vi "DPT Parse Debug Log.vi"(10 "text":string) -> (1 "Headers for Data":string[](array[string]), 2 "Array [raw rod, filt rod, outlet t, inlet t, coil, curve or hr]":i32[][](array[numeric]), 3 "Time Array":string[](array[string]))   [LabVIEW 2016]
panel:
  out "Numeric":i32
  out "Fault":i32
  out "Coil":i32
  out "Data Line":bool
  out "Time":string
  out "Line":string
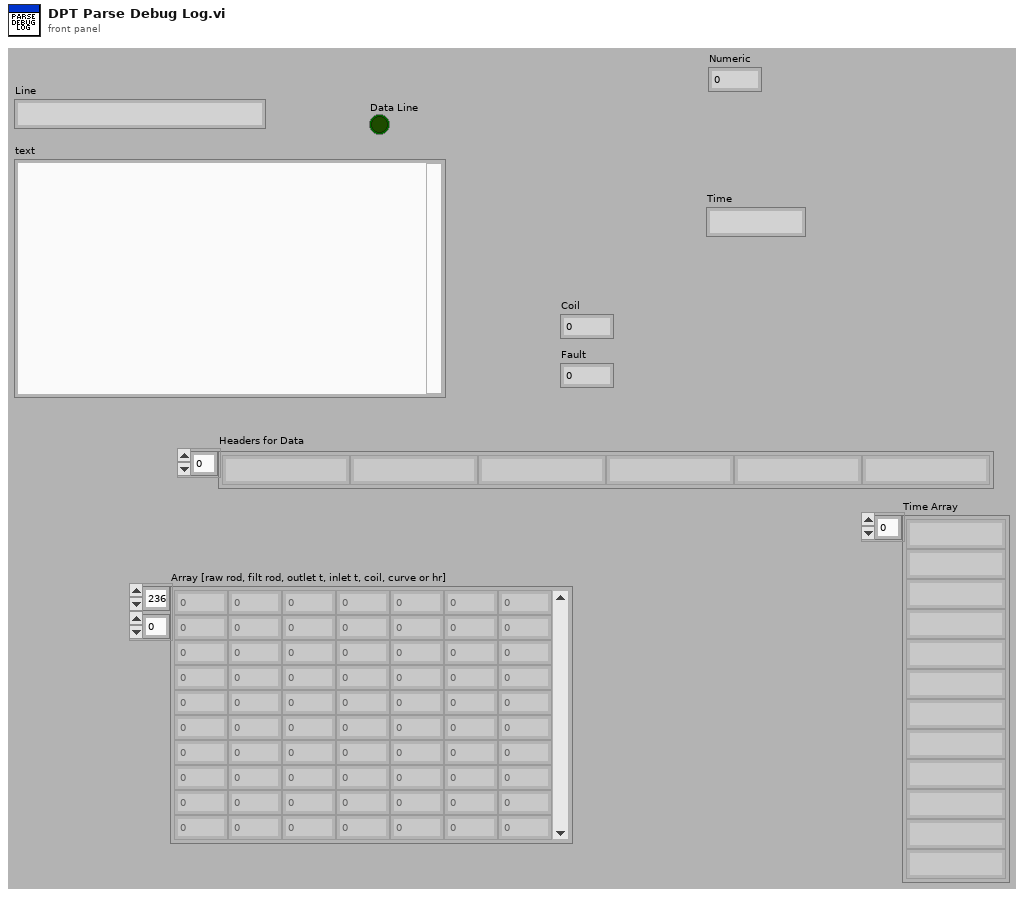
[diagram p1: front panel]
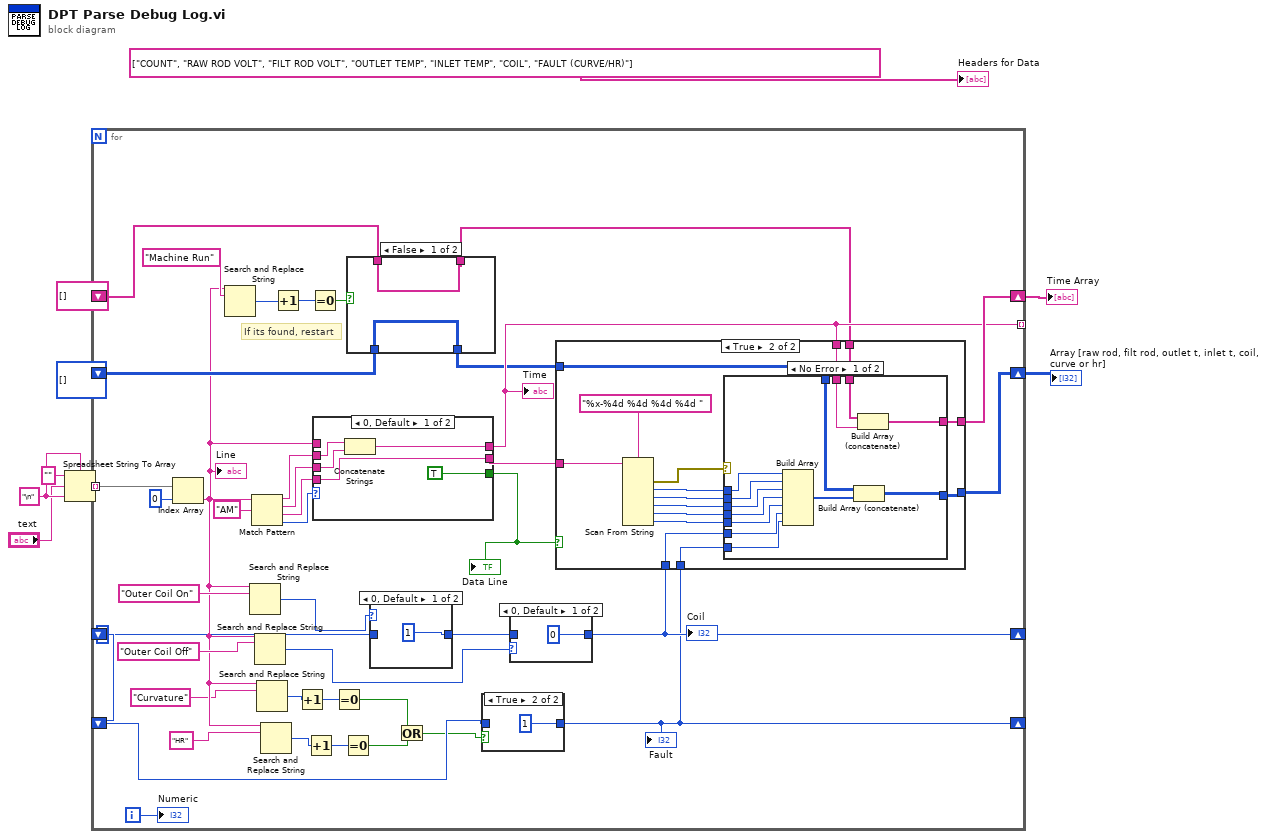
[diagram p0: block diagram]
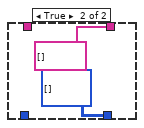
[diagram p5: hidden frame]
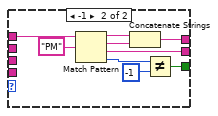
[diagram p8: hidden frame]
diagram:
  w4 = 0 ("output 5")
  w9 = "\n" ("delimiter (Tab)")
  n1 = Spreadsheet String To Array(delimiter (Tab)=w9, format string="", spreadsheet string="text", array type (2D Dbl)=w9) -> (array=w10:string[][])
  n2 = for {
    tunnel: w10 -> [w50] mode=indexing
    shift-right: [w11] -> w2
    shift-left: i32[][] [] -> [w34]
    tunnel: [w37] -> _ mode=indexing
    shift-right: [w38] -> w3
    shift-left: string[] [] -> [w32]
    shift-right: [w14] -> _
    shift-left: w4 -> [w23]
    shift-right: [w13] -> _
    shift-left: w4 -> [w22]
    i -> [w12]
    # "If its found, restart"
    n3 = Index Array(array=w50, index=0) -> (element=w29:string)
    "Line" <- w29
    n4 = Search and Replace String(input string=w29, search string="Machine Run") -> (number of replacements=w40:i32)  [unwired: 6 in, 3 out]
    n5 = Search and Replace String(input string=w29, search string="Outer Coil On") -> (number of replacements=w26:i32)  [unwired: 6 in, 3 out]
    n6 = Match Pattern(string=w29, regular expression="AM") -> (before substring=w46:string, match substring=w45:string, after substring=w43:string, offset past match=w47:i32)  [unwired: 1 in]
    n7 = Search and Replace String(input string=w29, search string="Outer Coil Off") -> (number of replacements=w25:i32)  [unwired: 6 in, 3 out]
    n8 = Search and Replace String(input string=w29, search string="Curvature") -> (number of replacements=w20:i32)  [unwired: 6 in, 3 out]
    n9 = Search and Replace String(input string=w29, search string="HR") -> (number of replacements=w18:i32)  [unwired: 6 in, 3 out]
    n10 = Increment(x=w40) -> (x+1=w39:i32)
    n11 = Increment(x=w20) -> (x+1=w21:i32)
    n12 = Increment(x=w18) -> (x+1=w19:i32)
    n13 = Equal To 0?(x=w39) -> (x = 0?=w36:bool)
    n14 = case shown="0, Default" w47 {
      tunnel: w46 -> [w97 _]
      tunnel: w45 -> [w96 _]
      tunnel: [w95 w102] -> w37
      tunnel: w29 -> [_ w106]
      tunnel: [TRUE w99] -> w44
      tunnel: [w93 w98] -> w42
      tunnel: w43 -> [w93 _]
      frame 0, Default {
        n15 = Concatenate Strings(w97, w96) -> (w95:string)
      }
      frame -1 {
        n16 = Match Pattern(string=w106, regular expression="PM") -> (before substring=w104:string, match substring=w103:string, after substring=w98:string, offset past match=w101:i32)  [unwired: 1 in]
        n17 = Concatenate Strings(w104, w103) -> (w102:string)
        n18 = Not Equal?(x=w101, y=-1 ("offset past match")) -> (x != y?=w99:bool)
      }
    }
    "Time" <- w37
    "Data Line" <- w44
    n19 = Equal To 0?(x=w21) -> (x = 0?=w17:bool)
    n20 = Equal To 0?(x=w19) -> (x = 0?=w16:bool)
    n21 = case shown="False" w36 {
      tunnel: [w58 i32[][] []] -> w35
      tunnel: w34 -> [w58 _]
      tunnel: [w57 string[] []] -> w33
      tunnel: w32 -> [w57 _]
      frame False {
      }
      frame True {
      }
    }
    n22 = case shown="0, Default" w26 {
      tunnel: [1 ("output 5") w56] -> w24
      tunnel: w23 -> [_ w56]
      frame 0, Default {
      }
      frame -1 {
      }
    }
    n23 = Or(x=w17, y=w16) -> (x .or. y?=w15:bool)
    n24 = case shown="True" w15 {
      tunnel: [w51 1 ("output 5")] -> w13
      tunnel: w22 -> [w51 _]
      frame False {
      }
      frame True {
      }
    }
    "Fault" <- w13
    n25 = case shown="0, Default" w25 {
      tunnel: [0 ("output 5") w54] -> w14
      tunnel: w24 -> [_ w54]
      frame 0, Default {
      }
      frame -1 {
      }
    }
    "Coil" <- w14
    n26 = case shown="True" w44 {
      tunnel: [w62 w68] -> w11
      tunnel: w35 -> [w62 w69]
      tunnel: w42 -> [_ w71]
      tunnel: [w61 w67] -> w38
      tunnel: w33 -> [w61 w66]
      tunnel: w37 -> [_ w65]
      tunnel: w14 -> [_ w64]
      tunnel: w13 -> [_ w63]
      frame False {
      }
      frame True {
        n27 = Scan From String(format string="%x-%4d %4d %4d %4d ", input string=w71) -> (error out=w70:errorcluster, output 1=w76:u32, output 2=w75:i32, output 3=w74:i32, output 4=w73:i32, output 5=w72:i32)  [unwired: 7 in, 2 out]
        n28 = case shown="No Error" w70 {
          tunnel: [w85 w91] -> w68
          tunnel: w76 -> [w90 _]
          tunnel: w75 -> [w89 _]
          tunnel: w74 -> [w88 _]
          tunnel: w73 -> [w87 _]
          tunnel: w72 -> [w86 _]
          tunnel: w69 -> [w83 w91]
          tunnel: [w82 w92] -> w67
          tunnel: w66 -> [w81 w92]
          tunnel: w65 -> [w80 _]
          tunnel: w64 -> [w79 _]
          tunnel: w63 -> [w78 _]
          frame No Error {
            n29 = Build Array(w90, w89, w88, w87, w86, w79, w78) -> (w84:u32[])
            n30 = Build Array (concatenate)(w83, w84) -> (w85:u32[][])
            n31 = Build Array (concatenate)(w81, w80) -> (w82:string[])
          }
          frame Error {
          }
        }
      }
    }
    "Numeric" <- w12
  }
  "Time Array" <- w3
  "Array [raw rod, filt rod, outlet t, inlet t, coil, curve or hr]" <- w2
  "Headers for Data" <- string[] ["COUNT", "RAW ROD VOLT", "FILT ROD VOLT", "OUTLET TEMP", "INLET TEMP", "COIL", "FAULT (CURVE/HR)"] ("Headers for Data")
